vi "Test MQTT-3.2.0-1.vi"(8 "error in (no error)":errorcluster) -> (0 "error out":errorcluster)   [LabVIEW 2013]
uses:
  <vilib>/LabVIEW Open Source Project/MQTT Control Packets/Control Packets/CONNACK/Connect Return Code -- enum.ctl
  <vilib>/LabVIEW Open Source Project/MQTT Control Packets/Control Packets/CONNACK/CONNACK.lvclass
  <vilib>/LabVIEW Open Source Project/MQTT Control Packets/Control Packets/CONNECT/CONNECT.lvclass
  <vilib>/LabVIEW Open Source Project/MQTT Control Packets/Control Packets/ControlPacket/ControlPacket.lvclass
  <vilib>/addons/_JKI Toolkits/Caraya/classes/Test/Test.lvclass
  <vilib>/addons/_JKI Toolkits/Caraya/classes/Assert/Assert.lvclass
  <vilib>/LabVIEW Open Source Project/MQTT Control Packets/Control Packets/DISCONNECT/DISCONNECT.lvclass
  <vilib>/LabVIEW Open Source Project/MQTT Connection/MQTT_Connection/Connection/Connection.lvclass
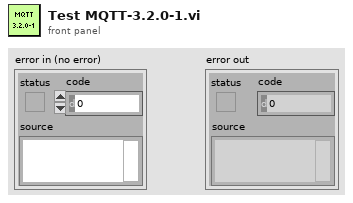
[diagram p1: front panel]
types:
  T1 = enum16{"Standard", "Buffered", "CRLF", "Immediate"}
  T2 = typedef "MQTT_Control_Packets.lvlib/CONNACK.lvclass/Connect Return Code -- enum.ctl" = enum16{"Connection accepted", "Unacceptable protocol version", "Identifier Rejected", "Server Unavailable", "Bad Username or Password", "Not Authorized"}
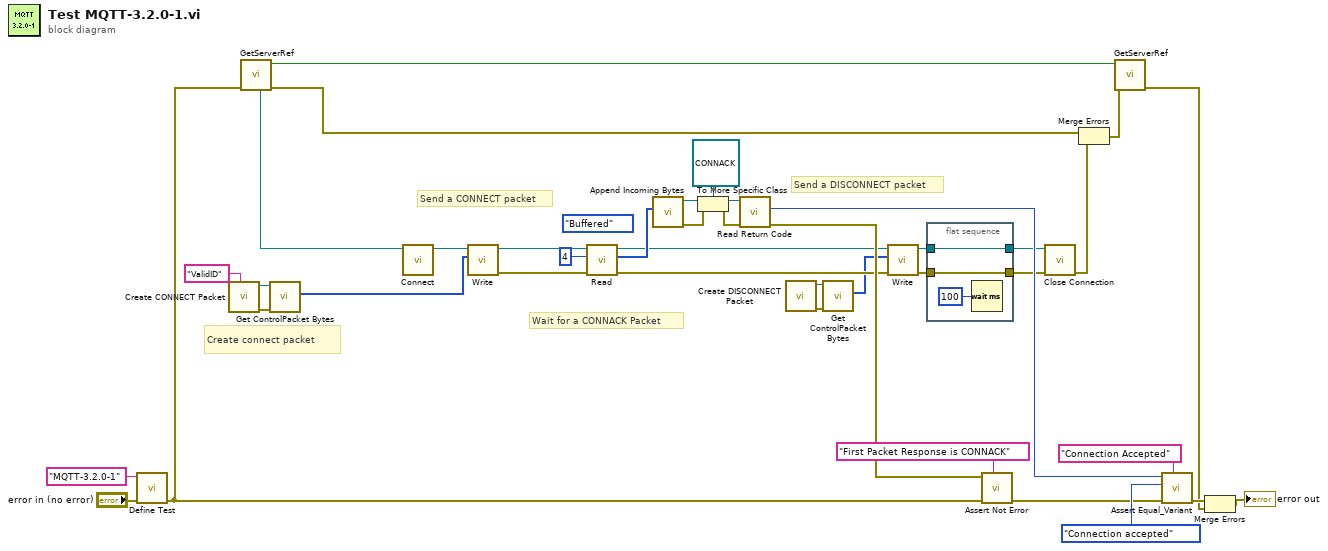
[diagram p0: block diagram]
diagram:
  (unwired) T1."Buffered" ("mode (standard)")
  # "Send a DISCONNECT packet"
  # "Wait for a CONNACK Packet"
  # "Create connect packet"
  # "Send a CONNECT packet"
  n1 = call <vilib>:"Define Test.vi"("error in (no error)"="error in (no error)", "Label (VI Title)"="MQTT-3.2.0-1") -> ("error out"=w20:errorcluster)  [unwired: 9 in]
  n2 = call <vilib>:"Create CONNECT Packet.vi"("Client ID (empty: generate new)"="ValidID") -> ("error out"=w39:errorcluster, "CONNECT"=w40:refnum<class "CONNECT.lvclass">)  [unwired: 8 in, 1 out]
  n3 = call "GetServerRef.vi"("error in"=w20) -> ("error out"=w17:errorcluster, "Created"=w21:bool, "Connection Config"=w2:refnum<class "Connection.lvclass">)  [unwired: 6 in, 2 out]
  n4 = call <vilib>:"Get ControlPacket Bytes.vi"("error in (no error)"=w39, "ControlPacket"=w40) -> ("Bytes Stream"=w15:u8[])  [unwired: 6 in, 3 out]
  n5 = call <vilib>:"Connect.vi"("Connection in"=w2) -> ("Connection out"=w1:refnum<class "Connection.lvclass">)  [unwired: 9 in, 1 out]
  n6 = call <vilib>:"Write.vi"("Bytes"=w15, "Connection in"=w1) -> ("error out"=w13:errorcluster, "Connection"=w14:refnum<class "Connection.lvclass">)  [unwired: 8 in]
  n7 = call <vilib>:"Read.vi"("error in (no error)"=w13, "bytes to read (100)"=4 ("bytes to read"), "TCPConnection in"=w14) -> ("error out"=w5:errorcluster, "Bytes"=w11:u8[], "TCPConnection out"=w7:refnum<class "Connection.lvclass">)  [unwired: 4 in, 2 out]
  n8 = call <vilib>:"Append Incoming Bytes.vi"("Incoming Packets"=w11) -> ("error out"=w23:errorcluster, "ControlPacket"=w31:refnum<class "ControlPacket.lvclass">)  [unwired: 7 in, 2 out]
  n9 = To More Specific Class(target class=refnum<class "CONNACK.lvclass"> refnum ("CONNACK in"), reference=w31, error in=w23) -> (specific class reference=w30:refnum<class "CONNACK.lvclass">, error out=w27:errorcluster)
  n10 = call <vilib>:"Read Return Code.vi"("error in (no error)"=w27, "CONNACK in"=w30) -> ("error out"=w25:errorcluster, "Return Code"=w29:T2)  [unwired: 7 in, 1 out]
  n11 = call <vilib>:"Create DISCONNECT Packet.vi"() -> ("error out"=w33:errorcluster, "DISCONNECT"=w32:refnum<class "DISCONNECT.lvclass">)  [unwired: 9 in, 1 out]
  n12 = call <vilib>:"Get ControlPacket Bytes.vi"("error in (no error)"=w33, "ControlPacket"=w32) -> ("Bytes Stream"=w3:u8[])  [unwired: 6 in, 3 out]
  n13 = call <vilib>:"Write.vi"("error in (no error)"=w5, "Bytes"=w3, "Connection in"=w7) -> ("error out"=w4:errorcluster, "Connection"=w6:refnum<class "Connection.lvclass">)  [unwired: 7 in]
  n14 = flat-sequence {
    tunnel: w6 -> [w43]
    tunnel: [w43] -> w10
    tunnel: [w41] -> w9
    tunnel: w4 -> [w41]
    frame #0 {
      n15 = Wait (ms)(milliseconds to wait=u32 100) -> ()  [unwired: 1 out]
    }
  }
  n16 = call <vilib>:"Assert Not Error.vi"("Label"="First Packet Response is CONNACK", "error in (no error)"=w20, "Not Error?"=w25) -> ("error out"=w26:errorcluster)  [unwired: 8 in]
  n17 = call <vilib>:"Close Connection.vi"("error in (no error)"=w9, "Connection in"=w10) -> ("error out"=w8:errorcluster)  [unwired: 8 in, 1 out]
  n18 = Merge Errors(w17, w8) -> (w18:errorcluster)
  n19 = call "GetServerRef.vi"("error in"=w18, "Destroy (F)"=w21) -> ("error out"=w19:errorcluster)  [unwired: 5 in, 4 out]
  n20 = call <vilib>:"Assert Equal_Variant.vi"("Label"="Connection Accepted", "error in (no error)"=w26, "Y"=Connect_Return_Code_--_enum."Connection accepted" ("Return Code"), "X"=w29) -> ("error out"=w37:errorcluster)  [unwired: 7 in]
  n21 = Merge Errors(w37, w19) -> (→"error out":errorcluster)
